vi "Get RPC VI template.vi"(8 "error in (no error)":errorcluster, 11 "Application in":refnum<vi>) -> (0 "error out":errorcluster, 2 "ProjectItem  reference out":refnum<vi>, 3 "Impl template RPC VI Reference":refnum<vi>)   [LabVIEW 2019, in "gRPC Template Creation Utility.lvlib"]
uses:
  gRPC Template Creation Utility.lvlib
  ServiceConstants.ctl
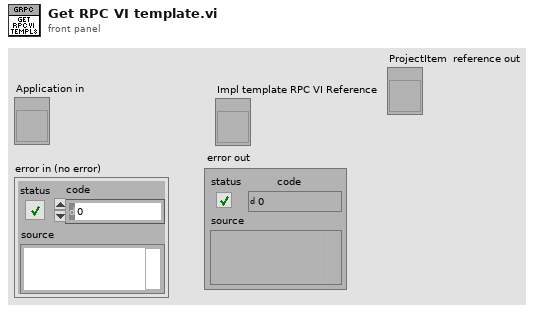
[diagram p1: front panel]
types:
  T1 = typedef "gRPC Template Creation Utility.lvlib/ServiceConstants.ctl" = enum16{"Stub", "Impl", "Usercode_server", "Generated_server", "RPC Service", "RPC Method package_service_method", "ServiceClass out", "ServiceClass in", "RPC Method"}
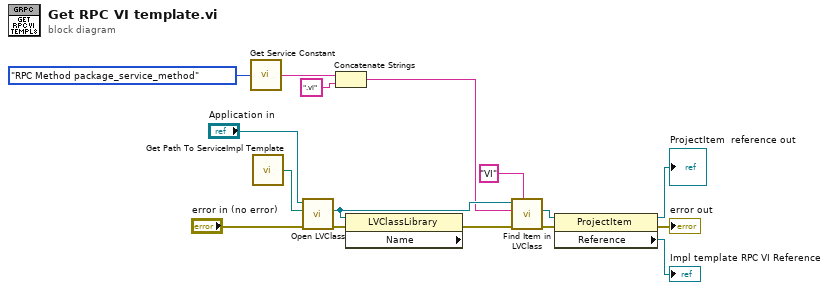
[diagram p0: block diagram]
diagram:
  n1 = call "Get Service Constant.vi"("Service Constant Strings"=ServiceConstants."RPC Method package_service_method") -> ("String Value"=w3:string)
  n2 = call "Get Path To ServiceImpl Template.vi"() -> ("appended path"=w10:path)
  n3 = call "Open LVClass.vi"("error in (no error)"="error in (no error)", "Full Path"=w10, "Application reference in"="Application in") -> ("error out"=w13:errorcluster, "LVClass out"=w12:refnum<vi>)  [unwired: 6 in, 1 out]
  n4 = Concatenate Strings(w3, ".vi" ("string")) -> (w1:string)
  n5 = property class="LVClassLibrary" props=["Name"](reference=w12, error in=w13) -> (error out=w14:errorcluster)  [unwired: 2 out]
  n6 = call "Find Item in LVClass.vi"("Item Type"="VI", "error in (no error)"=w14, "Item Name"=w1, "Class Item in"=w12) -> ("error out"=w15:errorcluster, "Project Item (Class Item)"=w16:refnum<vi>)  [unwired: 4 in, 2 out]
  n7 = property class="ProjectItem"(reference=w16, error in=w15) -> (reference out=→"ProjectItem  reference out":refnum<vi>, error out=→"error out":errorcluster, "Reference"=→"Impl template RPC VI Reference":refnum<vi>)
